vi "CSM - Set Log Filter Rules.vi"   [LabVIEW 2020, in "Communicable State Machine.lvlib"]
uses:
  Communicable State Machine.lvlib
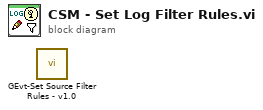
[diagram p0: block diagram]
diagram:
  n1 = call "GEvt-Set Source Filter Rules - v1.0.vi"() -> ()  [unwired: 11 in, 1 out]
